vi "FAHRENHEIT TO CELSIUS CONVERTER.vi"() -> ()   [LabVIEW 2020]
uses:
  <vilib>/express/express arith-compare/Formula/XNode/ExpressFormulaBlockNode.xnode
panel:
  out "Thermometer":dbl(slide) scale=0.0..100.0
  out "FORMULA C'":dbl
  out "EXPRESS NODE C'":dbl
  out "C'":dbl
  in  "F'":dbl
  # "FAHRENHEIT TO CELSIUS CONVERTER"
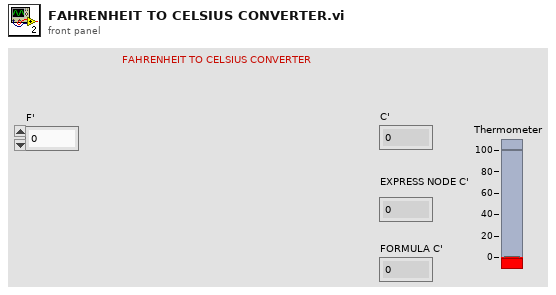
[diagram p1: front panel]
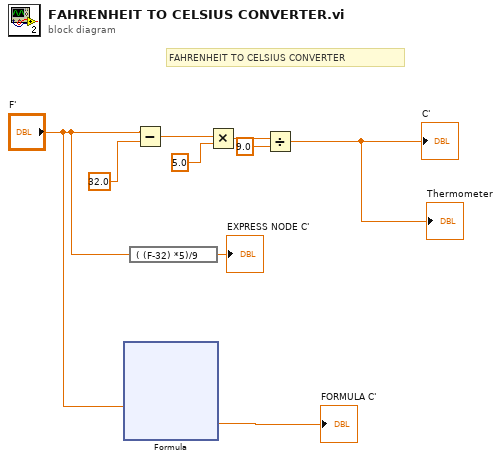
[diagram p0: block diagram]
diagram:
  # "FAHRENHEIT TO CELSIUS CONVERTER"
  n1 = xnode "Formula"("X1"="F'") -> ("Result"=→"FORMULA C'":dbl)  [unwired: 1 in, 1 out]
  n2 = expression code="( (F-32) *5)/9"("F'") -> (→"EXPRESS NODE C'":dbl)
  n3 = Subtract(x="F'", y=32.0 ("F'")) -> (x-y=w8:dbl)
  n4 = Multiply(x=w8, y=5.0) -> (x*y=w6:dbl)
  n5 = Divide(x=w6, y=9.0) -> (x/y=→"C'" →"Thermometer":dbl)
